vi "testingCameraSettings.vi"   [LabVIEW 2009, in "run.lvlib"]
uses:
  Hal/testing/run.lvlib
  CamaraSettings.lvclass
panel:
  # "runs the settings viewer"
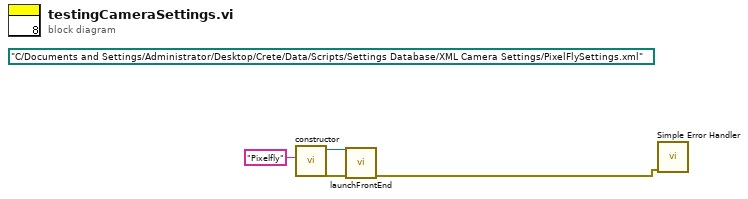
[diagram p0: block diagram]
diagram:
  (unwired) path "C:/Documents and Settings/Administrator/Desktop/Crete/Data/Scripts/Settings Database/XML Camera Settings/PixelFlySettings.xml"
  n1 = call "constructor.vi"("camera settings"="Pixelfly") -> ("error out"=w2:errorcluster, "CamaraSettings out"=w3:refnum<class "CamaraSettings.lvclass">)  [unwired: 9 in]
  n2 = call "launchFrontEnd.vi"("error in (no error)"=w2, "CamaraSettings in"=w3) -> ("error out"=w1:errorcluster)  [unwired: 8 in, 1 out]
  n3 = call <vilib>:"Simple Error Handler.vi"("error in (no error)"=w1) -> ()  [unwired: 4 in, 5 out]
